vi "Construct Event Keyword Filter.vi"(10 "Exclude Matches?":bool, 11 "Keywords":string[](array[string])) -> (3 "Event Keyword Filter out":refnum<class "Event Keyword Filter.lvclass">)   [LabVIEW 2017, in "Event Keyword Filter.lvclass"]
uses:
  Event Keyword Filter.lvclass
  Event Keyword Filter.lvclass/Event Keyword Filter.ctl
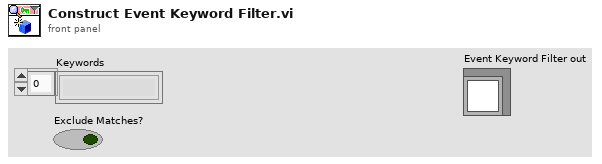
[diagram p1: front panel]
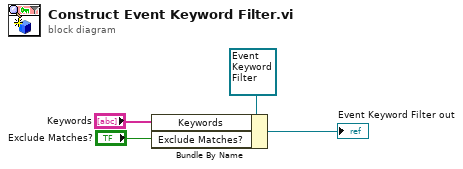
[diagram p0: block diagram]
diagram:
  n1 = Bundle By Name(cluster=refnum<class "Event Keyword Filter.lvclass"> refnum ("Event Keyword Filter in"), "Keywords"="Keywords", "Exclude Matches?"="Exclude Matches?") -> (→"Event Keyword Filter out":refnum<class "Event Keyword Filter.lvclass">)
